vi "Statistical Analysis.vi"(11 "value":map{i32, T1}(c390)) -> ()   [LabVIEW 2025, in "Full User Interface.lvlib"]
uses:
  Full User Interface.lvlib
  Station Info.ctl
  Test Unit/Test Unit.lvlib
panel:
  in  "Clear":bool
  out "Yields":dbl format="Yields: %.3f%%"
  out "Passed":u32 format="Passed: %d"
  out "Failed":u32 format="Failed: %d"
  out "Totals":u32 format="Totals: %d"
  out "2D Picture":picture
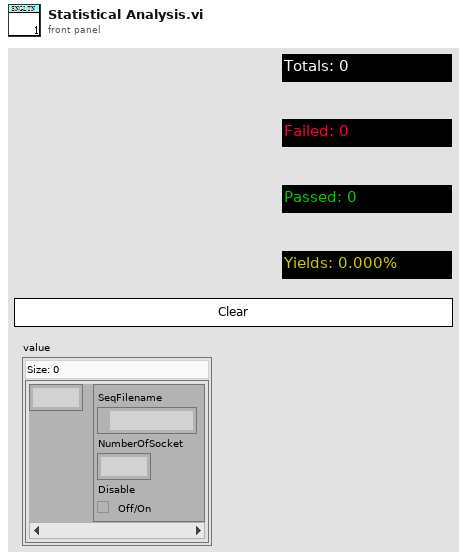
[diagram p1: front panel]
types:
  T1 = typedef "Full User Interface.lvlib/Station Info.ctl" = cluster{"SeqFilename":path, "NumberOfSocket":i32, "Disable":bool}
  T2 = cluster{"Width":u16, "Style":enum32{"Solid", "Dash", "Dot", "DashDot", "DashDotDot"}}
  T3 = cluster{"left":i16, "top":i16, "right":i16, "bottom":i16}
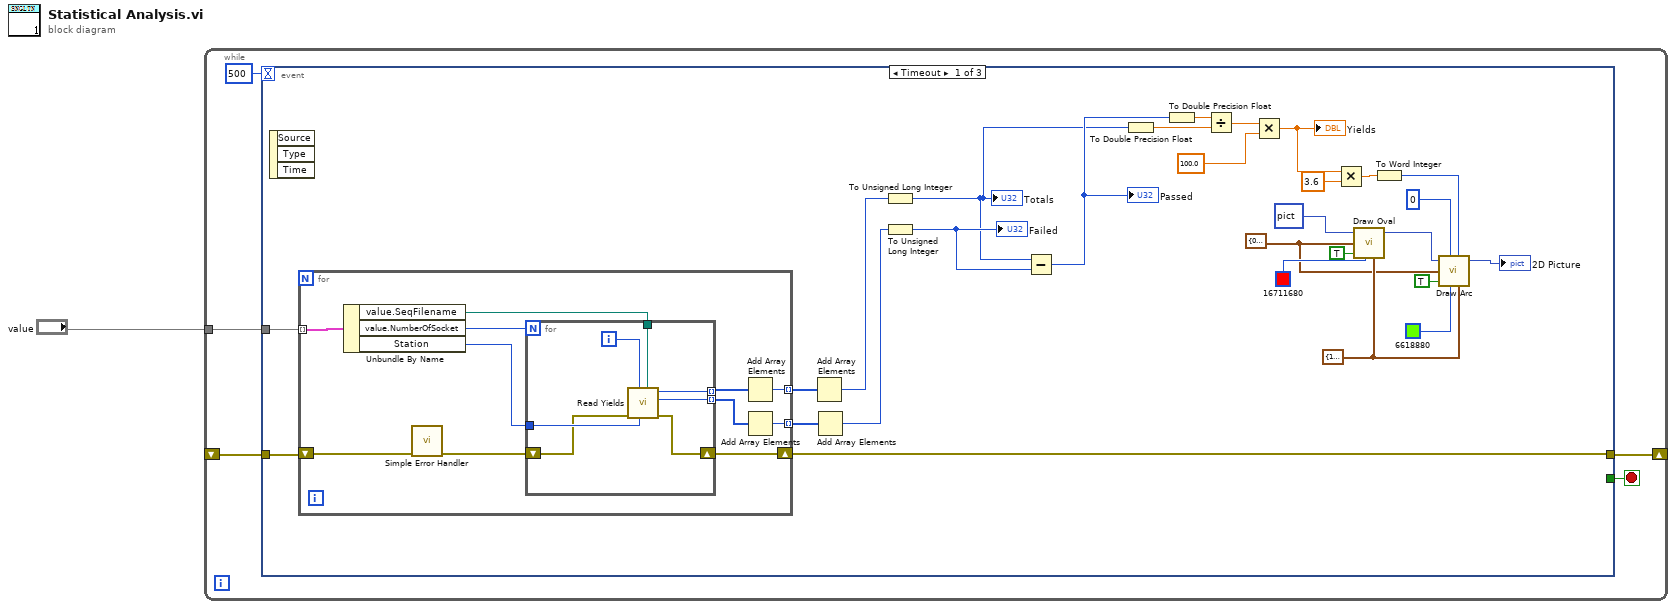
[diagram p0: block diagram]
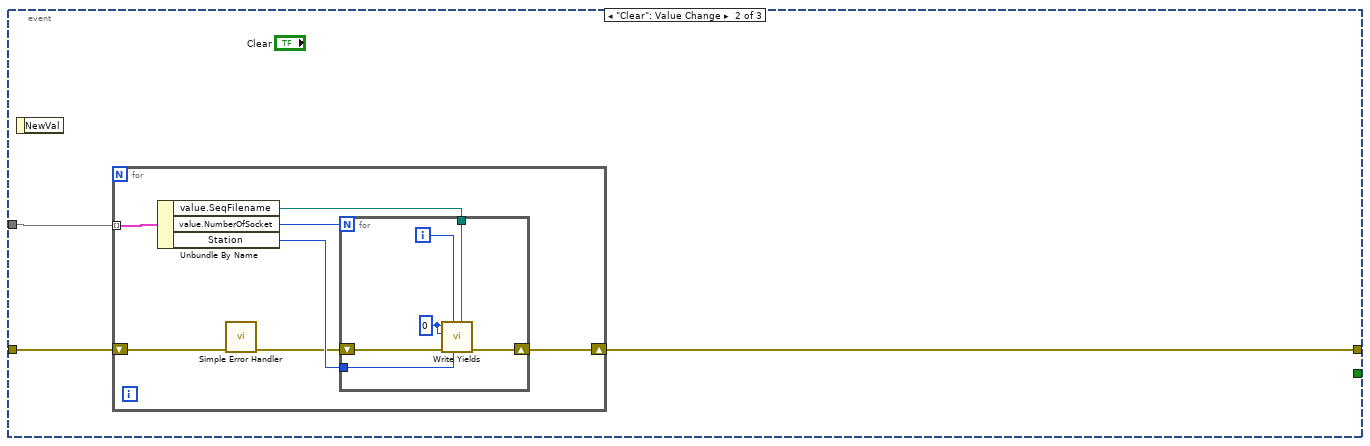
[diagram p2: hidden frame]
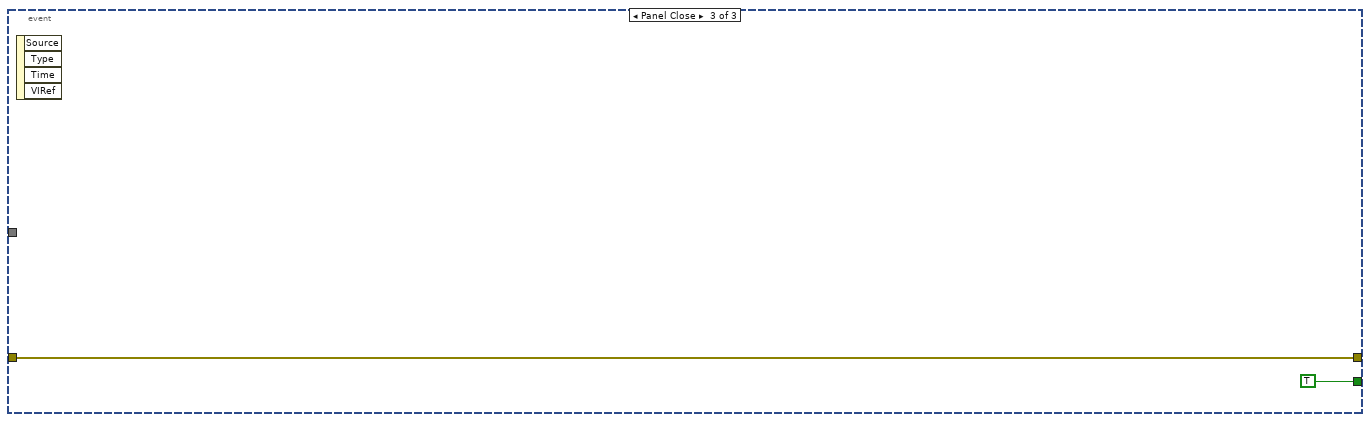
[diagram p3: hidden frame]
diagram:
  n1 = while {
    tunnel: "value" -> [w6]
    shift-right: [w3] -> _
    shift-left: _ -> [w2]
    stop <- w4 stop-if-true
    n2 = event shown="[0] Timeout" {
      selector: _ -> [_ _ _]
      dyn-events: _ -> [_ _ _]
      timeout: 500 -> [_ _ _]
      tunnel: w6 -> [w24 w55 _]
      tunnel: [_ _ TRUE] -> w4
      tunnel: [w7 w54 w69] -> w3
      tunnel: w2 -> [w8 w53 w69]
      event Timeout {
        w28 = T2 {"Width"=1, "Style"=enum."Solid"} ("pen")
        w27 = T3 {"left"=0, "top"=0, "right"=250, "bottom"=250} ("rect")
        n3 = event-data() -> ()  [unwired: 1 in, 3 out]
        n4 = for {
          tunnel: w24 -> [w45] mode=indexing
          tunnel: [w39] -> w23 mode=indexing
          tunnel: [w38] -> w22 mode=indexing
          shift-right: [w37] -> w7
          shift-left: w8 -> [w36]
          n5 = Unbundle By Name(w45) -> ("value.SeqFilename"=w42:path, "value.NumberOfSocket"=w44:i32, "Station"=w43:i32)
          n6 = call <vilib>:"Simple Error Handler.vi"("error in (no error)"=w36) -> ("error out"=w35:errorcluster)  [unwired: 4 in, 4 out]
          n7 = for {
            N: w44 -> [_]
            tunnel: w43 -> [w51]
            tunnel: w42 -> [w50]
            tunnel: [w49] -> w41 mode=indexing
            tunnel: [w48] -> w40 mode=indexing
            shift-right: [w47] -> w37
            shift-left: w35 -> [w46]
            i -> [w52]
            n8 = call "Read Yields.vi"("General.Sequence Path"=w50, "Station"=w51, "Socket"=w52, "error in (no error)"=w46) -> ("error out"=w47:errorcluster, "Failed"=w48:i32, "Totals"=w49:i32)  [unwired: 5 in]
          }
          n9 = Add Array Elements(numeric array=w41) -> (sum=w39:i32)
          n10 = Add Array Elements(numeric array=w40) -> (sum=w38:i32)
        }
        n11 = Add Array Elements(numeric array=w23) -> (sum=w20:i32)
        n12 = Add Array Elements(numeric array=w22) -> (sum=w19:i32)
        n13 = To Unsigned Long Integer(number=w20) -> (unsigned 32bit integer=w14:u32)
        "Totals" <- w14
        n14 = To Unsigned Long Integer(number=w19) -> (unsigned 32bit integer=w21:u32)
        "Failed" <- w21
        n15 = Subtract(x=w14, y=w21) -> (x-y=w15:u32)
        "Passed" <- w15
        n16 = To Double Precision Float(number=w14) -> (double precision float=w17:dbl)
        n17 = To Double Precision Float(number=w15) -> (double precision float=w18:dbl)
        n18 = Divide(x=w18, y=w17) -> (x/y=w16:dbl)
        n19 = Multiply(x=w16, y=100.0) -> (x*y=w12:dbl)
        "Yields" <- w12
        n20 = Multiply(x=w12, y=3.6) -> (x*y=w10:dbl)
        n21 = call <vilib>:"Draw Oval.vi"("picture"=picture data[5B], "rect"=w27, "fill?(F)"=TRUE, "color(black)"=u32 16711680, "pen"=w28) -> ("new picture"=w31:picture)  [unwired: 4 in]
        n22 = To Word Integer(number=w10) -> (16bit integer=w9:i16)
        n23 = call <vilib>:"Draw Arc.vi"("picture"=w31, "start angle[degrees]"=i16 0, "rect"=w27, "fill?(F)"=TRUE, "color(black)"=u32 6618880, "arc size[degrees]"=w9, "pen"=w28) -> ("new picture"=→"2D Picture":picture)  [unwired: 2 in]
      }
      event "Clear": Value Change {
        n24 = event-data() -> ()  [unwired: 1 in, 1 out]
        n25 = for {
          tunnel: w55 -> [w62] mode=indexing
          shift-right: [w58] -> w54
          shift-left: w53 -> [w57]
          n26 = Unbundle By Name(w62) -> ("value.SeqFilename"=w59:path, "value.NumberOfSocket"=w61:i32, "Station"=w60:i32)
          n27 = call <vilib>:"Simple Error Handler.vi"("error in (no error)"=w57) -> ("error out"=w56:errorcluster)  [unwired: 4 in, 4 out]
          n28 = for {
            N: w61 -> [_]
            tunnel: w60 -> [w63]
            tunnel: w59 -> [w65]
            shift-right: [w67] -> w58
            shift-left: w56 -> [w68]
            i -> [w66]
            w64 = 0 ("Totals")
            n29 = call "Write Yields.vi"("General.Sequence Path"=w65, "Station"=w63, "Socket"=w66, "error in (no error)"=w68, "Failed"=w64, "Totals"=w64) -> ("error out"=w67:errorcluster)  [unwired: 5 in]
          }
        }
      }
      event Panel Close {
        n30 = event-data() -> ()  [unwired: 1 in, 4 out]
      }
    }
  }
